vi "Array_Index_1D.vi"(6 "Error in (no error)":errorcluster, 10 "Array":string[](array[string]), 11 "Element string":string caption="Array string") -> (3 "Array row":i32, 4 "Error out":errorcluster)   [LabVIEW 2013]
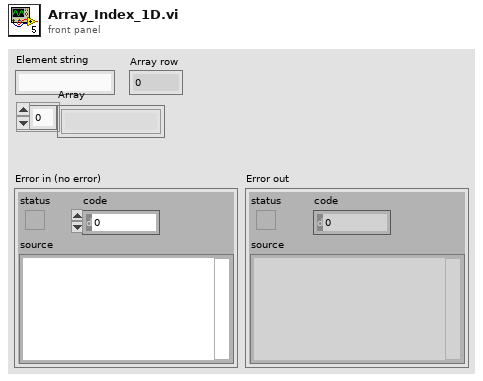
[diagram p1: front panel]
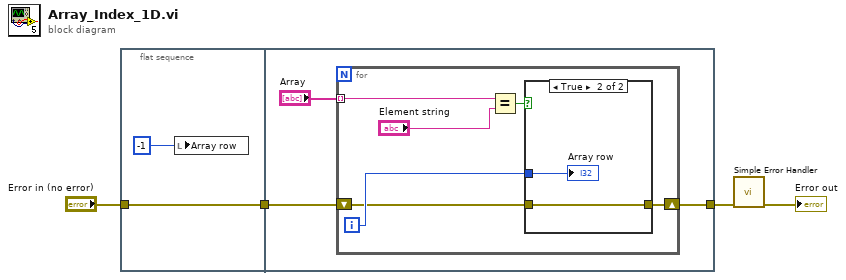
[diagram p0: block diagram]
diagram:
  n1 = flat-sequence {
    tunnel: "Error in (no error)" -> [w6]
    tunnel: [w6] -> w3
    tunnel: [w7] -> w2
    tunnel: w3 -> [w8]
    frame #0 {
      n2 = local write "Array row"(-1 ("VI index")) -> ()
    }
    frame #1 {
      n3 = for {
        shift-right: [w10] -> w7
        shift-left: w8 -> [w11]
        tunnel: "Array" -> [w13] mode=indexing
        i -> [w14]
        n4 = Equal?(x=w13, y="Element string") -> (x = y?=w15:bool)
        n5 = case shown="True" w15 {
          tunnel: w14 -> [_ w17]
          tunnel: w11 -> [w16 w18]
          tunnel: [w16 w18] -> w10
          frame False {
          }
          frame True {
            "Array row" <- w17
          }
        }
      }
    }
  }
  n6 = call <vilib>:"Simple Error Handler.vi"("error in (no error)"=w2) -> ("error out"=→"Error out":errorcluster)  [unwired: 4 in, 4 out]
